vi "ordina progressivo acq.vi"(11 "Curva in":string[][](array[string])) -> (3 "Curva 1":string[][](array[string]))   [LabVIEW 2019]
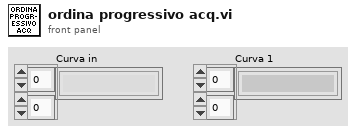
[diagram p1: front panel]
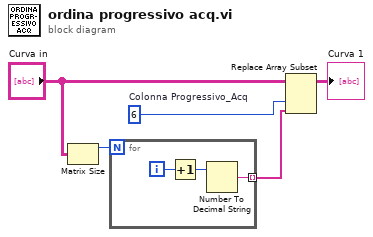
[diagram p0: block diagram]
diagram:
  w5 = 6  # Colonna Progressivo_Acq
  n1 = Matrix Size(0:"Curva in") -> (1:w1:i32)  [unwired: 1 out]
  n2 = for {
    N: w1 -> [_]
    tunnel: [w6] -> w2 mode=indexing
    i -> [w8]
    n3 = Increment(x=w8) -> (x+1=w7:i32)
    n4 = Number To Decimal String(number=w7) -> (decimal integer string=w6:string)  [unwired: 1 in]
  }
  n5 = Replace Array Subset(array="Curva in", new element=w2, index (col)=w5) -> (→"Curva 1":string[][])  [unwired: 1 in]
